vi "Shutdown.vi"(8 "error in (no error)":errorcluster, 11 "LoggerReference in":refnum<class "LoggerReference.lvclass">) -> (0 "error out":errorcluster)   [LabVIEW 2020, in "MVA Framework.lvlib" / "Composed Log.lvlib" / "LoggerReference.lvclass"]
uses:
  LoggerReference.lvclass
  LoggerReference.lvclass/LoggerReference.ctl
  Types/MessageCluster.ctl
  <vilib>/Utility/error.llb/Error Cluster From Error Code.vi
  Composed Log.lvlib
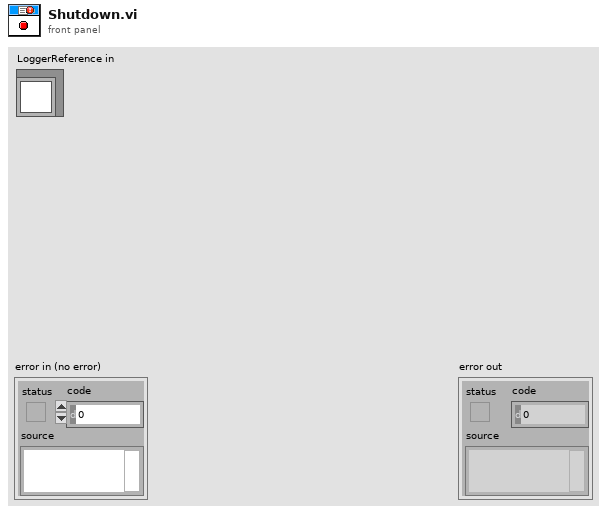
[diagram p1: front panel]
types:
  T1 = typedef "MVA Framework.lvlib/Composed Log.lvlib/MessageCluster.ctl" = cluster{"Message":string, "Data":variant}
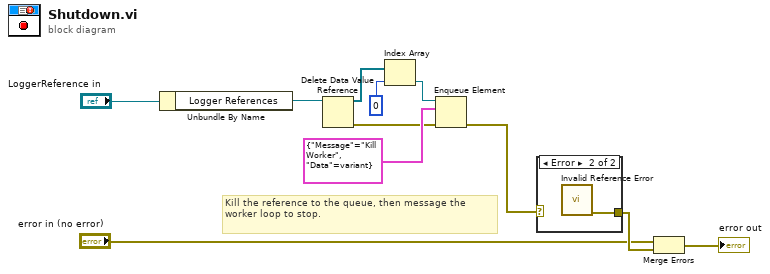
[diagram p0: block diagram]
diagram:
  # "Kill the reference to the queue, then message the worker loop to stop."
  n1 = Unbundle By Name("LoggerReference in") -> ("Logger References"=w7:refnum<data-value>)
  n2 = Delete Data Value Reference(data value reference=w7) -> (data value=w3:refnum<queue>[], error out=w5:errorcluster)  [unwired: 1 in]
  n3 = Index Array(array=w3, index=0) -> (element=w1:refnum<queue>)
  n4 = Enqueue Element(queue=w1, element=T1 {"Message"="Kill Worker", "Data"=variant}, error in (no error)=w5) -> (error out=w4:errorcluster)  [unwired: 1 in, 2 out]
  n5 = case shown="Error" w4 {
    selector: w4 -> [w12 _]
    tunnel: [w12 w13] -> w11
    frame No Error {
    }
    frame Error {
      n6 = call "Invalid Reference Error.vi"() -> ("error out"=w13:errorcluster)  [unwired: 11 in]
    }
  }
  n7 = Merge Errors("error in (no error)", w11) -> (→"error out":errorcluster)
